vi "Intensity Graph Horizontal Linecut.vi"(8 "error in (no error)":errorcluster, 9 "width (horizontal)":dbl, 10 "Intensity Data":dbl[][](array[numeric]), 11 "graph_utilities in":refnum<class "graph_utilities.lvclass">) -> (0 "error out":errorcluster, 2 "XY-data horizontal":cluster{"Intensity Data":dbl[], "Array":dbl[]}, 3 "graph_utilities out":refnum<class "graph_utilities.lvclass">)   [LabVIEW 2016, in "graph_utilities.lvclass"]
uses:
  graph_utilities.lvclass
  graph_utilities.lvclass/graph_utilities.ctl
  <vilib>/Analysis/baseanly.llb/A x Vector.vi
  <vilib>/Analysis/NI_AALBase.lvlib
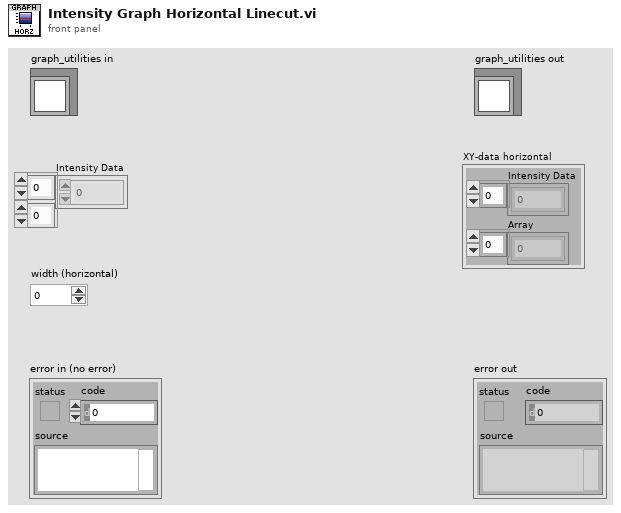
[diagram p1: front panel]
types:
  T1 = typedef "LVPointDoubleTypeDef.ctl" = cluster{"Cursor X":dbl, "Cursor Y":dbl}
  T2 = typedef "LVOffsetAndMultiplierTypeDef.ctl" = cluster{"Offset":dbl, "Multiplier":dbl}
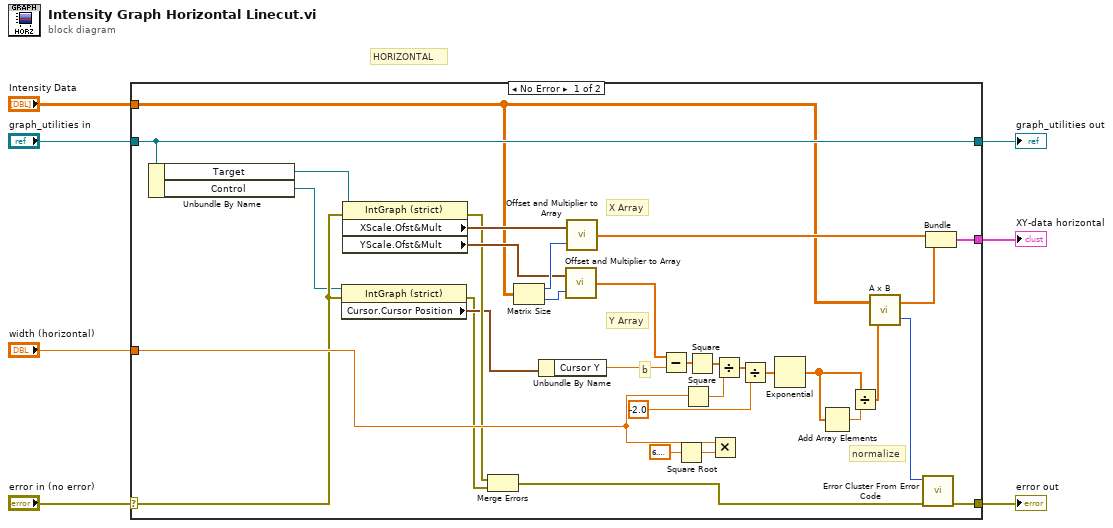
[diagram p0: block diagram]
diagram:
  # "HORIZONTAL"
  n1 = case shown="No Error" "error in (no error)" {
    selector: "error in (no error)" -> [w12 w41]
    tunnel: [w14 w41] -> w6
    tunnel: [w39 w40] -> w4
    tunnel: "graph_utilities in" -> [w39 w40]
    tunnel: "Intensity Data" -> [w16 _]
    tunnel: [w38 _] -> w2
    tunnel: "width (horizontal)" -> [w20 _]
    frame No Error {
      # "normalize"
      # "b"
      # "X Array"
      # "Y Array"
      n2 = Unbundle By Name(w39) -> ("Target"=w11:refnum<vi>, "Control"=w10:refnum<vi>)
      n3 = property on="Property Node" class="IntGraph (strict)"(reference=w10, error in=w12) -> (error out=w8:errorcluster, "Cursor.Cursor Position"=w13:T1)  [unwired: 1 out]
      n4 = property on="Property Node" class="IntGraph (strict)"(reference=w11, error in=w12) -> (error out=w15:errorcluster, "XScale.Ofst&Mult"=w35:T2, "YScale.Ofst&Mult"=w34:T2)  [unwired: 1 out]
      n5 = Merge Errors(w15, w8) -> (w9:errorcluster)
      n6 = Matrix Size(0:w16) -> (1:w37:i32, 2:w36:i32)
      n7 = Unbundle By Name(w13) -> ("Cursor Y"=w21:dbl)
      n8 = call "Offset and Multiplier to Array.vi"("Size"=w36, "Offset and Multiplier"=w34) -> ("Array"=w22:dbl[])
      n9 = call "Offset and Multiplier to Array.vi"("Size"=w37, "Offset and Multiplier"=w35) -> ("Array"=w19:dbl[])
      n10 = Subtract(x=w22, y=w21) -> (x-y=w32:dbl[])
      n11 = Square Root(x=6.283185307179586) -> (sqrt(x)=w29:dbl)
      n12 = Square(x=w20) -> (x^2=w28:dbl)
      n13 = Square(x=w32) -> (x^2=w31:dbl[])
      n14 = Multiply(x=w20, y=w29) -> ()  [unwired: 1 out]
      n15 = Divide(x=w31, y=w28) -> (x/y=w27:dbl[])
      n16 = Divide(x=w27, y=-2.0 ("value")) -> (x/y=w25:dbl[])
      n17 = Exponential(1:w25) -> (0:w23:dbl[])
      n18 = Add Array Elements(numeric array=w23) -> (sum=w24:dbl)
      n19 = Divide(x=w23, y=w24) -> (x/y=w33:dbl[])
      n20 = call-poly <vilib>:"A x B.vi"("Vector"=w33, "A"=w16) -> ("error"=w17:i32, "A x Vector"=w18:dbl[])
      n21 = call <vilib>:"Error Cluster From Error Code.vi"("error in (no error)"=w9, "error code (0)"=w17) -> ("error out"=w14:errorcluster)  [unwired: 7 in]
      n22 = Bundle("Array"=w19, "A x Vector"=w18) -> (w38:cluster{"Array":dbl[], "A x Vector":dbl[]})  [unwired: 1 in]
    }
    frame Error {
    }
  }
  "error out" <- w6
  "graph_utilities out" <- w4
  "XY-data horizontal" <- w2
